vi "Get Station Firmware Version V.vi"(8 "error in (no error)":errorcluster, 11 "verSt":string) -> (0 "error out":errorcluster, 2 "function return":i16, 3 "verSt out":string)   [LabVIEW 2009, in "VantagePro.lvlib"]
doc: "DllAccess short int _stdcall GetStationFirmwareVersion_V ( char *verSt);"
uses:
  VantagePro.lvlib
  <userlib>/VantagePro/VantagePro.dll
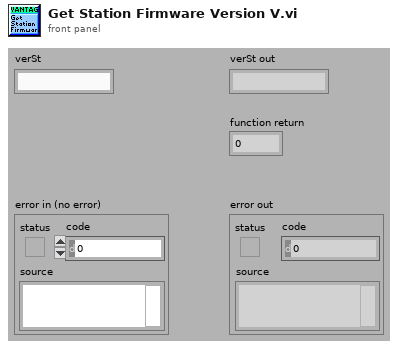
[diagram p1: front panel]
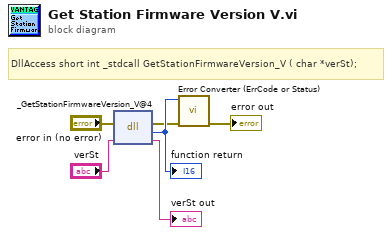
[diagram p0: block diagram]
diagram:
  # "DllAccess short int _stdcall GetStationFirmwareVersion_V ( char *verSt);"
  n1 = dll-call lib="C:/Program Files/National Instruments/LabVIEW 2010/user.lib/VantagePro/VantagePro.*" fn="_GetStationFirmwareVersion_V@4"(error in="error in (no error)", "verSt"="verSt") -> (error out=w2:errorcluster, w6:i16, "verSt"=→"verSt out":string)  [unwired: 2 in, 1 out]
  "function return" <- w6
  n2 = call "Error Converter (ErrCode or Status).vi"("error in (no error)"=w2, "error code"=w6) -> ("error out"=→"error out":errorcluster)  [unwired: 9 in]
